vi "pmu_Build Data Block.vi"(5 "init meas data":u8[](array[numeric]), 6 "digitals":u16[](array[numeric]), 7 "STAT field":u16, 8 "analogs byte array":u8[](array[numeric]), 9 "dfreq byte array":u8[](array[numeric]), 10 "freq byte array":u8[](array[numeric]), 11 "phasor byte array":u8[](array[numeric])) -> (3 "data block":u8[](array[numeric]))   [LabVIEW 2013, in "NI_EP_PMU.lvlib"]
uses:
  <vilib>/addons/Electrical Power/PMU/NI_EP_PMU.lvlib
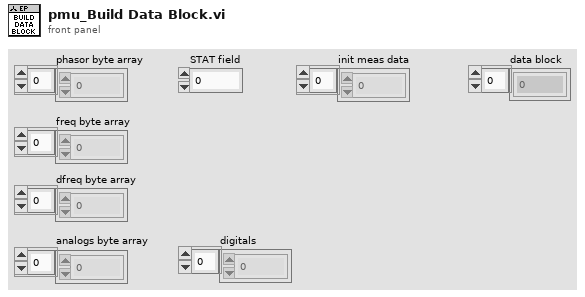
[diagram p1: front panel]
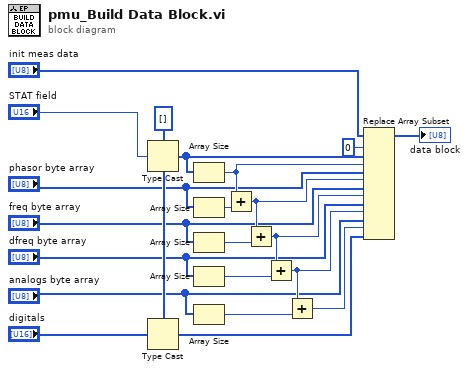
[diagram p0: block diagram]
diagram:
  w10 = u8[] [] ("appended array")
  n1 = Type Cast(type=w10, x="STAT field") -> (*(type *) &x=w20:u8[])
  n2 = Type Cast(type=w10, x="digitals") -> (*(type *) &x=w9:u8[])
  n3 = Array Size(array=w20) -> (size(s)=w18:i32)
  n4 = Array Size(array="phasor byte array") -> (size(s)=w19:i32)
  n5 = Array Size(array="freq byte array") -> (size(s)=w17:i32)
  n6 = Array Size(array="dfreq byte array") -> (size(s)=w15:i32)
  n7 = Array Size(array="analogs byte array") -> (size(s)=w13:i32)
  n8 = Add(x=w18, y=w19) -> (x+y=w16:i32)
  n9 = Add(x=w16, y=w17) -> (x+y=w14:i32)
  n10 = Add(x=w14, y=w15) -> (x+y=w12:i32)
  n11 = Add(x=w12, y=w13) -> (x+y=w11:i32)
  n12 = Replace Array Subset(array="init meas data", new element #1=w20, index #1=0 ("index"), new element #2="phasor byte array", index #2=w18, new element #3="freq byte array", index #3=w16, new element #4="dfreq byte array", index #4=w14, new element #5="analogs byte array", index #5=w12, new element #6=w9, index #6=w11) -> (→"data block":u8[])
